vi "addVariantToBSONDocument.vi"(8 "error in (no error)":errorcluster, 10 "Variant":variant, 11 "tBSONDocument in":refnum<class "tBSONDocument.lvclass">) -> (0 "error out":errorcluster, 3 "tBSONDocument out":refnum<class "tBSONDocument.lvclass">)   [LabVIEW 2013, in "BSON.lvlib" / "tBSONDocument.lvclass"]
uses:
  tBSONDocument.lvclass
  status.ctl
  addI32Element.vi
  addI64Element.vi
  addDoubleElement.vi
  addBooleanElement.vi
  addStringElement.vi
  addTimestampElement.vi
  addDocumentElement.vi
  addI32[]Element.vi
  addI64[]Element.vi
  addDouble[]Element.vi
  addBoolean[]Element.vi
  addString[]Element.vi
  addTimestamp[]Element.vi
  addDocument[]Element.vi
  <vilib>/Utility/VariantDataType/VariantType.lvlib
  BSON.lvlib
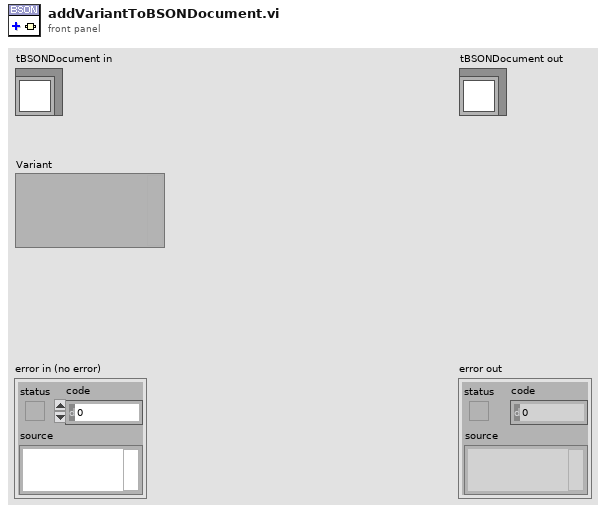
[diagram p1: front panel]
types:
  T1 = typedef "BSON.lvlib/status.ctl" = enum16{"Stream Corrupted or Ended Abruptly", "Incorrect Type In Stream", "ObjectID Invalid", "Method Not Implemented", "Invalid Name", "Invalid URI", "AutoReconnect", "Operation Failed", "Incorrectly Configured", "Cursor Not Found", "Timeout", "Invalid Type", "Empty Name", "Duplicate Name", "MD5Incorrect"}
  T2 = typedef "VariantType.lvlib/Type.ctl" = enum8{"Invalid Type", "Void", "I8", "I16", "I32", "I64", "U8", "U16", "U32", "U64", "Single Float", "Double Float", "Extended Float", "Single Complex", "Double Complex", "Extended Complex", "Enum U8", "Enum U16", "Enum U32", "Enum U64", "Single Float With Unit", "Double Float With Unit", "Extended Float With Unit", "Single Complex with Unit", "Double Complex with Unit", "Extended Complex with Unit", "Boolean", "String", "Path", "Picture", "Tag", "Array", "Cluster", "Variant", "LV Variant", "Waveform", "Timestamp", "Digital Waveform", "Digital Data", "ExpressData", "Refnum", "External Data", "VI", "Poly VI", "LabVIEW Class Instance", "Fixed Point"}
  T3 = typedef "VariantType.lvlib/MemoryInfo.ctl" = cluster{"Type":T4, "Size":u32}
  T4 = typedef "VariantType.lvlib/MemoryType.ctl" = enum16{"Variable", "Fixed", "Bounded"}
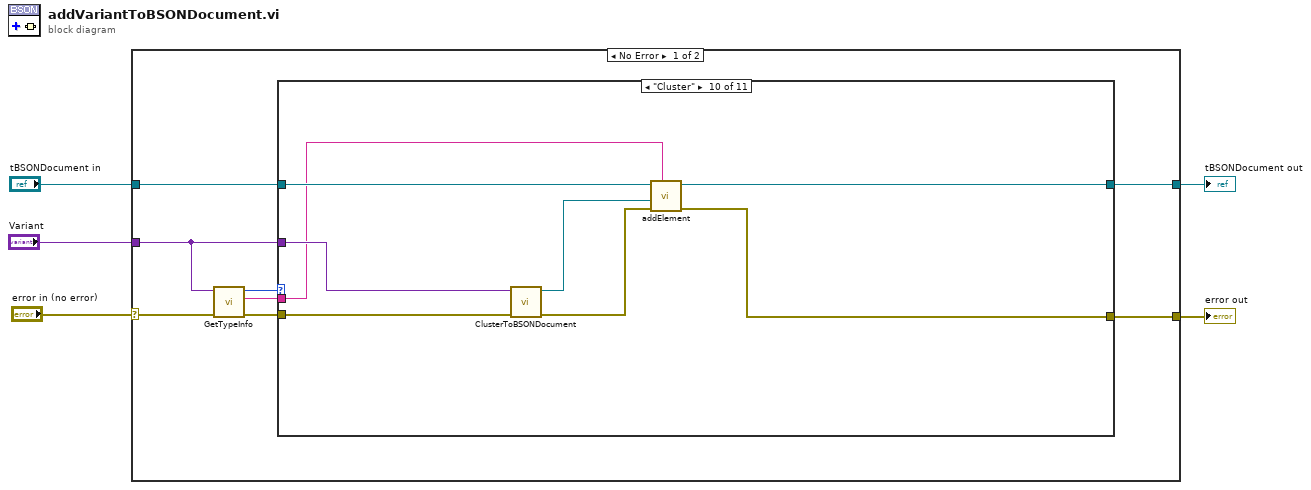
[diagram p0: block diagram]
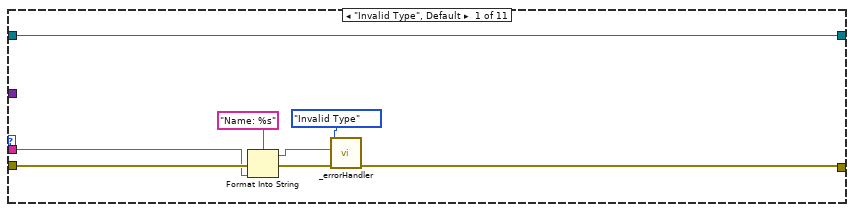
[diagram p2: hidden frame]
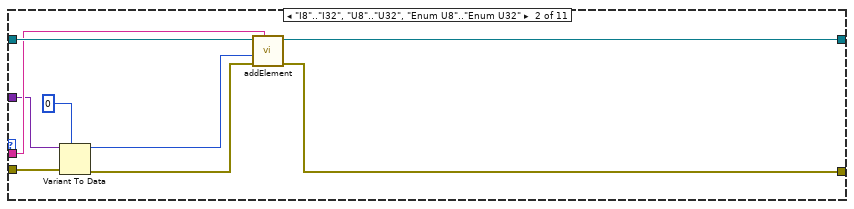
[diagram p3: hidden frame]
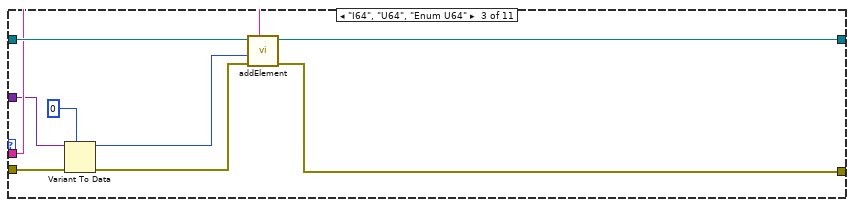
[diagram p4: hidden frame]
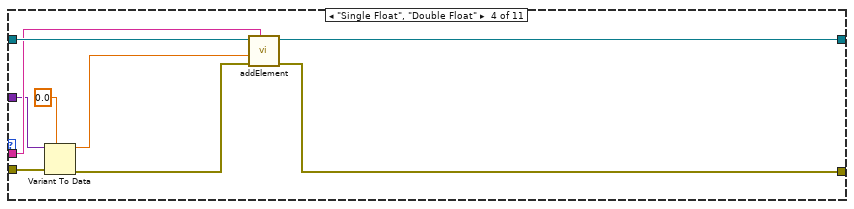
[diagram p5: hidden frame]
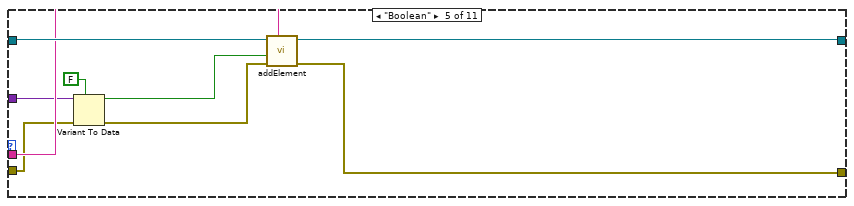
[diagram p6: hidden frame]
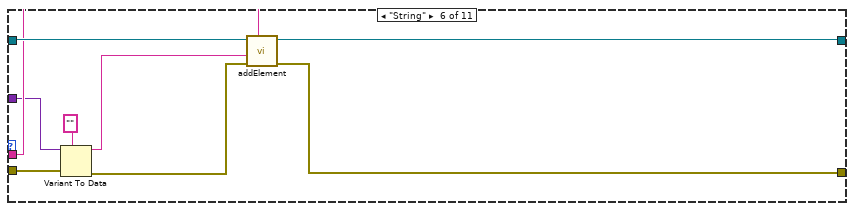
[diagram p7: hidden frame]
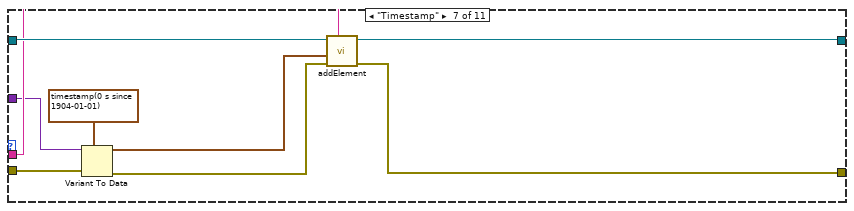
[diagram p8: hidden frame]
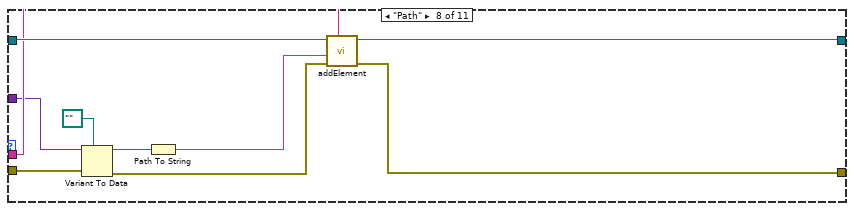
[diagram p9: hidden frame]
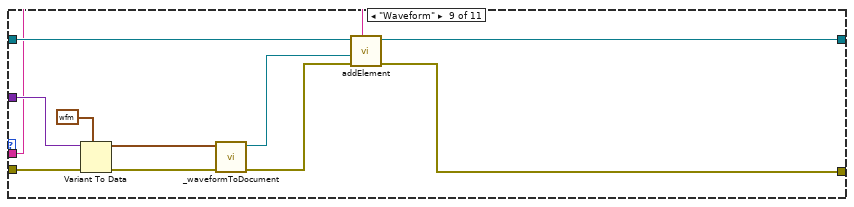
[diagram p10: hidden frame]
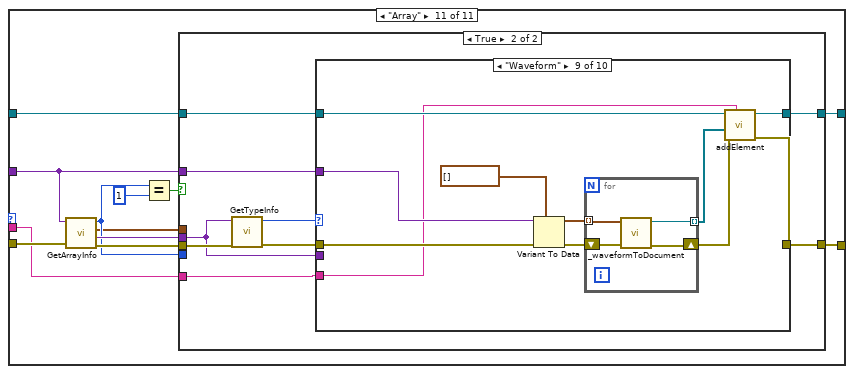
[diagram p11: hidden frame]
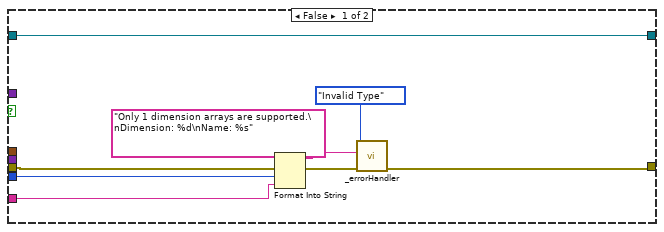
[diagram p12: hidden frame]
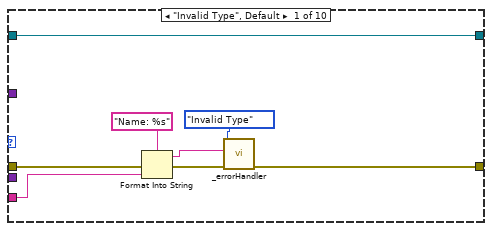
[diagram p13: hidden frame]
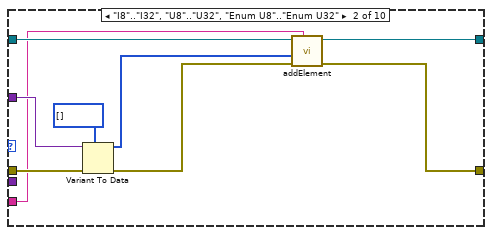
[diagram p14: hidden frame]
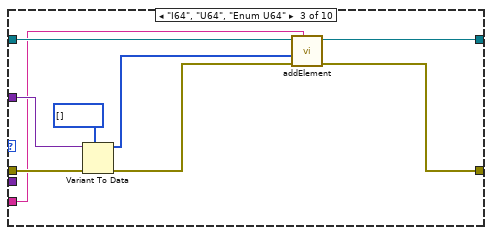
[diagram p15: hidden frame]
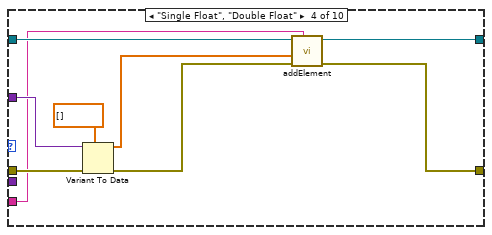
[diagram p16: hidden frame]
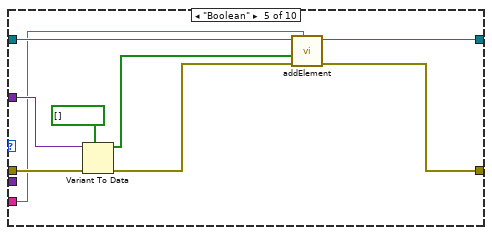
[diagram p17: hidden frame]
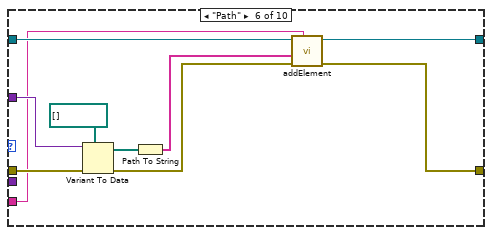
[diagram p18: hidden frame]
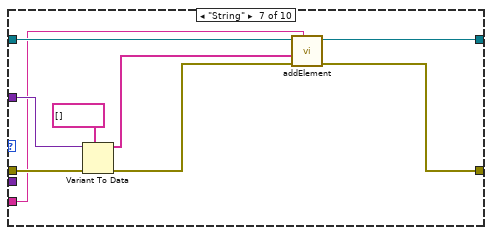
[diagram p19: hidden frame]
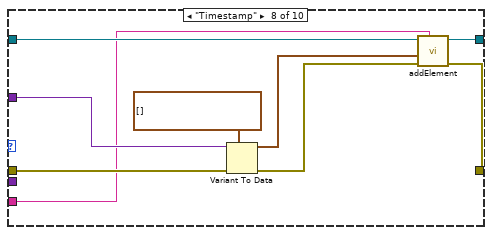
[diagram p20: hidden frame]
diagram:
  n1 = case shown="No Error" "error in (no error)" {
    selector: "error in (no error)" -> [w9 w239]
    tunnel: [w7 w239] -> w4
    tunnel: [w8 w238] -> w2
    tunnel: "tBSONDocument in" -> [w10 w238]
    tunnel: "Variant" -> [w6 _]
    frame No Error {
      n2 = call <vilib>:"GetTypeInfo.vi"("error in (no error)"=w9, "Variant"=w6) -> ("error out"=w11:errorcluster, "Name"=w12:string, "Type Enum"=w13:T2)  [unwired: 5 in, 2 out]
      n3 = case shown="\"Cluster\"" w13 {
        tunnel: w10 -> [w21 w29 w38 w48 w57 w65 w75 w85 w91 w102 w111]
        tunnel: [w19 w27 w33 w42 w54 w60 w70 w81 w89 w99 w112] -> w7
        tunnel: [w21 w26 w34 w47 w55 w61 w71 w82 w90 w98 w109] -> w8
        tunnel: w12 -> [w14 w24 w37 w46 w56 w62 w72 w83 w88 w97 w113]
        tunnel: w11 -> [w18 w23 w32 w41 w53 w59 w69 w80 w96 w103 w116]
        tunnel: w6 -> [_ w22 w31 w40 w52 w58 w68 w79 w95 w104 w110]
        frame "Invalid Type", Default {
          n4 = Format Into String(format string="Name: %s", error in=w18, w14) -> (resulting string=w16:string, error out=w17:errorcluster)  [unwired: 1 in]
          n5 = call "_errorHandler.vi"("error in (no error)"=w17, "Additional Text"=w16, "Error Type"=status."Invalid Type") -> ("error out"=w19:errorcluster)  [unwired: 8 in]
        }
        frame "I8".."I32", "U8".."U32", "Enum U8".."Enum U32" {
          n6 = Variant To Data(error in=w23, type=0, Variant=w22) -> (data=w25:i32, error out=w28:errorcluster)
          n7 = call-poly "addElement.vi"("Name"=w24, "error in (no error)"=w28, "Value"=w25, "tBSONDocument in"=w29) -> ("error out"=w27:errorcluster, "tBSONDocument out"=w26:refnum<class "tBSONDocument.lvclass">)  [unwired: 6 in]
        }
        frame "I64", "U64", "Enum U64" {
          n8 = Variant To Data(error in=w32, type=i64 0, Variant=w31) -> (data=w35:i64, error out=w36:errorcluster)
          n9 = call-poly "addElement.vi"("Name"=w37, "error in (no error)"=w36, "Value"=w35, "tBSONDocument in"=w38) -> ("error out"=w33:errorcluster, "tBSONDocument out"=w34:refnum<class "tBSONDocument.lvclass">)  [unwired: 6 in]
        }
        frame "Single Float", "Double Float" {
          n10 = Variant To Data(error in=w41, type=0.0, Variant=w40) -> (data=w44:dbl, error out=w43:errorcluster)
          n11 = call-poly "addElement.vi"("Name"=w46, "error in (no error)"=w43, "Value"=w44, "tBSONDocument in"=w48) -> ("error out"=w42:errorcluster, "tBSONDocument out"=w47:refnum<class "tBSONDocument.lvclass">)  [unwired: 6 in]
        }
        frame "Boolean" {
          n12 = Variant To Data(error in=w53, type=FALSE, Variant=w52) -> (data=w51:bool, error out=w50:errorcluster)
          n13 = call-poly "addElement.vi"("Name"=w56, "error in (no error)"=w50, "Value"=w51, "tBSONDocument in"=w57) -> ("error out"=w54:errorcluster, "tBSONDocument out"=w55:refnum<class "tBSONDocument.lvclass">)  [unwired: 6 in]
        }
        frame "String" {
          n14 = Variant To Data(error in=w59, type="", Variant=w58) -> (data=w63:string, error out=w64:errorcluster)
          n15 = call-poly "addElement.vi"("Name"=w62, "error in (no error)"=w64, "Value"=w63, "tBSONDocument in"=w65) -> ("error out"=w60:errorcluster, "tBSONDocument out"=w61:refnum<class "tBSONDocument.lvclass">)  [unwired: 6 in]
        }
        frame "Timestamp" {
          n16 = Variant To Data(error in=w69, type=timestamp(0 s since 1904-01-01), Variant=w68) -> (data=w73:timestamp, error out=w74:errorcluster)
          n17 = call-poly "addElement.vi"("Name"=w72, "error in (no error)"=w74, "Value"=w73, "tBSONDocument in"=w75) -> ("error out"=w70:errorcluster, "tBSONDocument out"=w71:refnum<class "tBSONDocument.lvclass">)  [unwired: 6 in]
        }
        frame "Path" {
          n18 = Variant To Data(error in=w80, type=path "", Variant=w79) -> (data=w77:path, error out=w84:errorcluster)
          n19 = Path To String(path=w77) -> (string=w76:string)
          n20 = call-poly "addElement.vi"("Name"=w83, "error in (no error)"=w84, "Value"=w76, "tBSONDocument in"=w85) -> ("error out"=w81:errorcluster, "tBSONDocument out"=w82:refnum<class "tBSONDocument.lvclass">)  [unwired: 6 in]
        }
        frame "Waveform" {
          n21 = Variant To Data(error in=w96, type=waveform(dbl) {"t0"=timestamp(0 s since 1904-01-01), "dt"=1.0, "Y"=[]} ("waveform"), Variant=w95) -> (data=w93:waveform(dbl), error out=w92:errorcluster)
          n22 = call "_waveformToDocument.vi"("error in (no error)"=w92, "waveform"=w93) -> ("error out"=w86:errorcluster, "tBSONDocument out"=w87:refnum<class "tBSONDocument.lvclass">)  [unwired: 8 in]
          n23 = call-poly "addElement.vi"("Name"=w88, "error in (no error)"=w86, "Value"=w87, "tBSONDocument in"=w91) -> ("error out"=w89:errorcluster, "tBSONDocument out"=w90:refnum<class "tBSONDocument.lvclass">)  [unwired: 6 in]
        }
        frame "Cluster" {
          n24 = call "ClusterToBSONDocument.vi"("error in (no error)"=w103, "Variant"=w104) -> ("error out"=w100:errorcluster, "tBSONDocument out"=w101:refnum<class "tBSONDocument.lvclass">)  [unwired: 8 in]
          n25 = call-poly "addElement.vi"("Name"=w97, "error in (no error)"=w100, "Value"=w101, "tBSONDocument in"=w102) -> ("error out"=w99:errorcluster, "tBSONDocument out"=w98:refnum<class "tBSONDocument.lvclass">)  [unwired: 6 in]
        }
        frame "Array" {
          n26 = call <vilib>:"GetArrayInfo.vi"("error in (no error)"=w116, "Variant"=w110) -> ("error out"=w115:errorcluster, "ArrayElement"=w114:variant, "Array Lengths"=w105:T3[], "NDims"=w108:i32)  [unwired: 6 in]
          n27 = Equal?(x=w108, y=1) -> (x = y?=w106:bool)
          n28 = case shown="True" w106 {
            tunnel: w115 -> [w121 w134]
            tunnel: w114 -> [_ w127]
            tunnel: w113 -> [w120 w131]
            tunnel: [w118 w130] -> w112
            tunnel: w111 -> [w117 w129]
            tunnel: w110 -> [_ w128]
            tunnel: w108 -> [w119 _]
            tunnel: [w117 w126] -> w109
            tunnel: w105 -> [_ _]
            frame False {
              n29 = Format Into String(format string="Only 1 dimension arrays are supported.\nDimension: %d\nName: %s", error in=w121, w119, w120) -> (resulting string=w123:string, error out=w124:errorcluster)  [unwired: 1 in]
              n30 = call "_errorHandler.vi"("error in (no error)"=w124, "Additional Text"=w123, "Error Type"=status."Invalid Type") -> ("error out"=w118:errorcluster)  [unwired: 8 in]
            }
            frame True {
              n31 = call <vilib>:"GetTypeInfo.vi"("error in (no error)"=w134, "Variant"=w127) -> ("error out"=w133:errorcluster, "Type Enum"=w132:T2)  [unwired: 5 in, 3 out]
              n32 = case shown="\"Waveform\"" w132 {
                tunnel: w133 -> [w138 w151 w160 w169 w178 w188 w197 w206 w217 w227]
                tunnel: w131 -> [w137 w143 w152 w161 w170 w181 w189 w198 w211 w228]
                tunnel: [w136 w145 w154 w163 w172 w183 w191 w200 w213 w230] -> w130
                tunnel: w129 -> [w135 w148 w157 w166 w175 w185 w194 w203 w214 w233]
                tunnel: w128 -> [_ w150 w159 w168 w177 w187 w196 w205 w216 w226]
                tunnel: [w135 w144 w153 w162 w171 w182 w190 w199 w212 w229] -> w126
                tunnel: w127 -> [_ _ _ _ _ _ _ _ _ w225]
                frame "Invalid Type", Default {
                  n33 = Format Into String(format string="Name: %s", error in=w138, w137) -> (resulting string=w140:string, error out=w141:errorcluster)  [unwired: 1 in]
                  n34 = call "_errorHandler.vi"("error in (no error)"=w141, "Additional Text"=w140, "Error Type"=status."Invalid Type") -> ("error out"=w136:errorcluster)  [unwired: 8 in]
                }
                frame "I8".."I32", "U8".."U32", "Enum U8".."Enum U32" {
                  n35 = Variant To Data(error in=w151, type=i32[] [], Variant=w150) -> (data=w146:i32[], error out=w147:errorcluster)
                  n36 = call-poly "addElement.vi"("Name"=w143, "error in (no error)"=w147, "Value"=w146, "tBSONDocument in"=w148) -> ("error out"=w145:errorcluster, "tBSONDocument out"=w144:refnum<class "tBSONDocument.lvclass">)  [unwired: 6 in]
                }
                frame "I64", "U64", "Enum U64" {
                  n37 = Variant To Data(error in=w160, type=i64[] [], Variant=w159) -> (data=w155:i64[], error out=w156:errorcluster)
                  n38 = call-poly "addElement.vi"("Name"=w152, "error in (no error)"=w156, "Value"=w155, "tBSONDocument in"=w157) -> ("error out"=w154:errorcluster, "tBSONDocument out"=w153:refnum<class "tBSONDocument.lvclass">)  [unwired: 6 in]
                }
                frame "Single Float", "Double Float" {
                  n39 = Variant To Data(error in=w169, type=dbl[] [], Variant=w168) -> (data=w164:dbl[], error out=w165:errorcluster)
                  n40 = call-poly "addElement.vi"("Name"=w161, "error in (no error)"=w165, "Value"=w164, "tBSONDocument in"=w166) -> ("error out"=w163:errorcluster, "tBSONDocument out"=w162:refnum<class "tBSONDocument.lvclass">)  [unwired: 6 in]
                }
                frame "Boolean" {
                  n41 = Variant To Data(error in=w178, type=bool[] [], Variant=w177) -> (data=w173:bool[], error out=w174:errorcluster)
                  n42 = call-poly "addElement.vi"("Name"=w170, "error in (no error)"=w174, "Value"=w173, "tBSONDocument in"=w175) -> ("error out"=w172:errorcluster, "tBSONDocument out"=w171:refnum<class "tBSONDocument.lvclass">)  [unwired: 6 in]
                }
                frame "Path" {
                  n43 = Variant To Data(error in=w188, type=path[] [], Variant=w187) -> (data=w180:path[], error out=w184:errorcluster)
                  n44 = Path To String(path=w180) -> (string=w179:string[])
                  n45 = call-poly "addElement.vi"("Name"=w181, "error in (no error)"=w184, "Value"=w179, "tBSONDocument in"=w185) -> ("error out"=w183:errorcluster, "tBSONDocument out"=w182:refnum<class "tBSONDocument.lvclass">)  [unwired: 6 in]
                }
                frame "String" {
                  n46 = Variant To Data(error in=w197, type=string[] [], Variant=w196) -> (data=w192:string[], error out=w193:errorcluster)
                  n47 = call-poly "addElement.vi"("Name"=w189, "error in (no error)"=w193, "Value"=w192, "tBSONDocument in"=w194) -> ("error out"=w191:errorcluster, "tBSONDocument out"=w190:refnum<class "tBSONDocument.lvclass">)  [unwired: 6 in]
                }
                frame "Timestamp" {
                  n48 = Variant To Data(error in=w206, type=timestamp[] [], Variant=w205) -> (data=w201:timestamp[], error out=w202:errorcluster)
                  n49 = call-poly "addElement.vi"("Name"=w198, "error in (no error)"=w202, "Value"=w201, "tBSONDocument in"=w203) -> ("error out"=w200:errorcluster, "tBSONDocument out"=w199:refnum<class "tBSONDocument.lvclass">)  [unwired: 6 in]
                }
                frame "Waveform" {
                  n50 = Variant To Data(error in=w217, type=waveform(dbl)[] [], Variant=w216) -> (data=w209:waveform(dbl)[], error out=w210:errorcluster)
                  n51 = for {
                    shift-right: [w219] -> w207
                    shift-left: w210 -> [w221]
                    tunnel: w209 -> [w220] mode=indexing
                    tunnel: [w218] -> w208 mode=indexing
                    n52 = call "_waveformToDocument.vi"("error in (no error)"=w221, "waveform"=w220) -> ("error out"=w219:errorcluster, "tBSONDocument out"=w218:refnum<class "tBSONDocument.lvclass">)  [unwired: 8 in]
                  }
                  n53 = call-poly "addElement.vi"("Name"=w211, "error in (no error)"=w207, "Value"=w208, "tBSONDocument in"=w214) -> ("error out"=w213:errorcluster, "tBSONDocument out"=w212:refnum<class "tBSONDocument.lvclass">)  [unwired: 6 in]
                }
                frame "Cluster" {
                  n54 = Build Array(w225) -> (w224:variant[])
                  n55 = Variant To Data(error in=w227, type=w224, Variant=w226) -> (data=w223:variant[], error out=w222:errorcluster)
                  n56 = for {
                    shift-right: [w237] -> w231
                    shift-left: w222 -> [w234]
                    tunnel: [w236] -> w232 mode=indexing
                    tunnel: w223 -> [w235] mode=indexing
                    n57 = call "ClusterToBSONDocument.vi"("error in (no error)"=w234, "Variant"=w235) -> ("error out"=w237:errorcluster, "tBSONDocument out"=w236:refnum<class "tBSONDocument.lvclass">)  [unwired: 8 in]
                  }
                  n58 = call-poly "addElement.vi"("Name"=w228, "error in (no error)"=w231, "Value"=w232, "tBSONDocument in"=w233) -> ("error out"=w230:errorcluster, "tBSONDocument out"=w229:refnum<class "tBSONDocument.lvclass">)  [unwired: 6 in]
                }
              }
            }
          }
        }
      }
    }
    frame Error {
    }
  }
  "error out" <- w4
  "tBSONDocument out" <- w2
